vi "ex_CreateColHdngs.vi"(1 "col heading labels":string[](array[string]), 4 "all col heading data":string[][](array[string])) -> (0 "final col headings":string[][](array[string]))   [LabVIEW 2020]
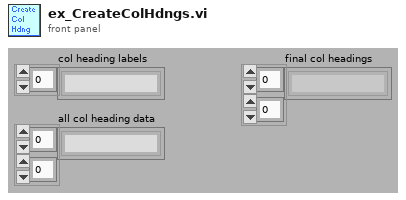
[diagram p1: front panel]
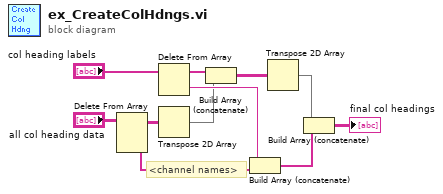
[diagram p0: block diagram]
diagram:
  # "<channel names>"
  n1 = Delete From Array(array="all col heading data") -> (deleted portion=w7:string[], array with subset deleted=w3:string[][])  [unwired: 3 in]
  n2 = Delete From Array(array="col heading labels") -> (deleted portion=w5:string, array with subset deleted=w8:string[])  [unwired: 2 in]
  n3 = Transpose 2D Array(2D array=w3) -> (transposed array=w2:string[][])
  n4 = Build Array (concatenate)(w8, w2) -> (w11:string[][])
  n5 = Build Array (concatenate)(w5, w7) -> (w6:string[])
  n6 = Transpose 2D Array(2D array=w11) -> (transposed array=w4:string[][])
  n7 = Build Array (concatenate)(w4, w6) -> (→"final col headings":string[][])
